vi "AD5781StandaloneTest.vi"() -> ()   [LabVIEW 2014]
uses:
  <vilib>/rvi/interface/nirviOpenFPGA/nirviOpenFPGA.xnode
  FPGA Bitfiles/TiTaProj_DAF_AD5781Standalone_V1.lvbitx
  <vilib>/rvi/interface/nirviReadWriteControl/nirviReadWriteControl.xnode
  <vilib>/rvi/interface/Simulation/niFpgaSimulationCallBeginRW.vi
  <vilib>/rvi/errors/niLvFpgaAdjustHostInterfaceError.vi
  <vilib>/rvi/interface/nirviCloseFPGA/nirviCloseFPGA.xnode
  <vilib>/FPGAPlugInAG/PXI-7852R/niLvFpga_Open_PXI-7852R.vi
  <vilib>/rvi/interface/common/dynamic/niFpgaDynamicAddResources.vi
  <vilib>/FPGAPlugInAG/Dynamic/niLvFpga_Close_Dynamic.vi
panel:
  in  "stop":bool
  in  "setDACRegister":u32 format="%024b"
  in  "setVolt":bool
  out "DacState":enum16{"init", "idle", "setVolt", "error"}(ring)
  out "actDACRegister":u32 format="%024b"
  out "DacStateCmdByHost":enum16{"init", "idle", "setVolt", "error"}(ring)
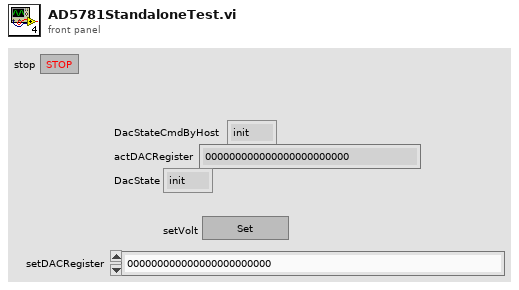
[diagram p1: front panel]
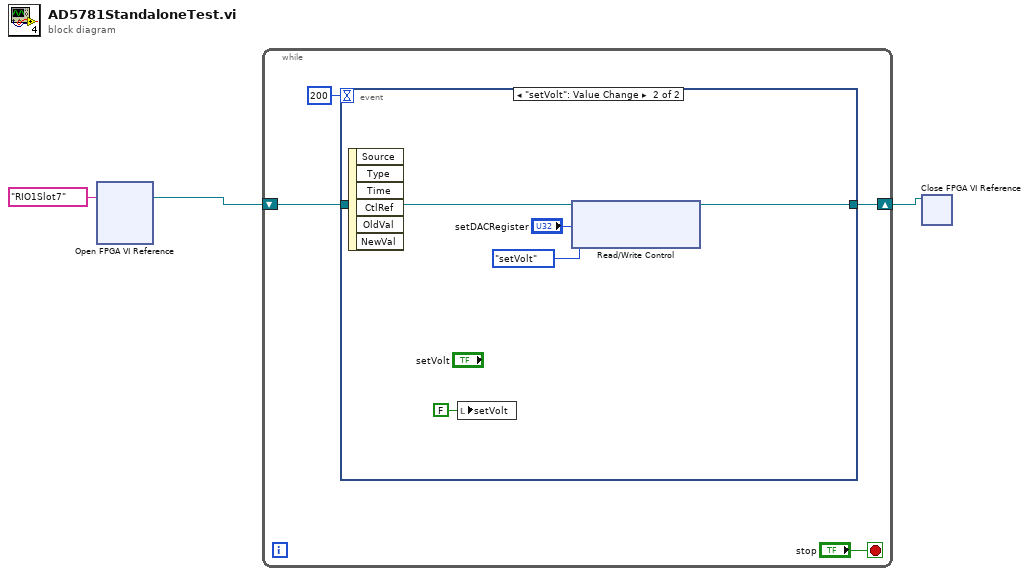
[diagram p0: block diagram]
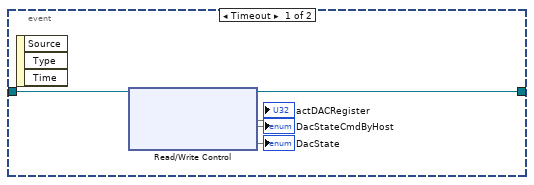
[diagram p2: hidden frame]
diagram:
  n1 = xnode "Open FPGA VI Reference"("resource name"=tag "RIO1Slot7") -> ("FPGA VI Reference Out"=w1:refnum<k20>)  [unwired: 1 in, 1 out]
  n2 = while {
    shift-right: [w7] -> w2
    shift-left: w1 -> [w6]
    stop <- "stop" stop-if-true
    n3 = event shown="[1] \"setVolt\": Value Change" {
      selector: _ -> [_ _]
      dyn-events: _ -> [_ _]
      timeout: 200 -> [_ _]
      tunnel: [w8 w15] -> w7
      tunnel: w6 -> [w9 w16]
      event Timeout {
        n4 = event-data() -> ()  [unwired: 1 in, 3 out]
        n5 = xnode "Read/Write Control"("FPGA VI Reference In"=w9) -> ("FPGA VI Reference Out"=w8:refnum<k20>, "DacStateCmdByHost"=→"DacStateCmdByHost", "actDACRegister"=→"actDACRegister", "DacState"=→"DacState")  [unwired: 1 in, 1 out]
      }
      event "setVolt": Value Change {
        n6 = event-data() -> ()  [unwired: 1 in, 6 out]
        n7 = local write "setVolt"(FALSE ("setVolt")) -> ()
        n8 = xnode "Read/Write Control"("FPGA VI Reference In"=w16, "setDACRegister"="setDACRegister", "DacStateCmdByHost"=enum16{"init", "idle", "setVolt", "error"}."setVolt") -> ("FPGA VI Reference Out"=w15:refnum<k20>)  [unwired: 1 in, 1 out]
      }
    }
  }
  n9 = xnode "Close FPGA VI Reference"("FPGA VI Reference In"=w2) -> ()  [unwired: 1 in, 1 out]
